vi "簡單狀態機.vi"() -> ()   [LabVIEW 2021]
panel:
  out "震幅":string
  out "頻率":string
  out "Waveform Graph":dbl[](graph)
  in  "Next Button":bool
  in  "Save Button":bool
  in  "Open Button":bool
  in  "Stop Button":bool
  in  "Cancel Button":bool
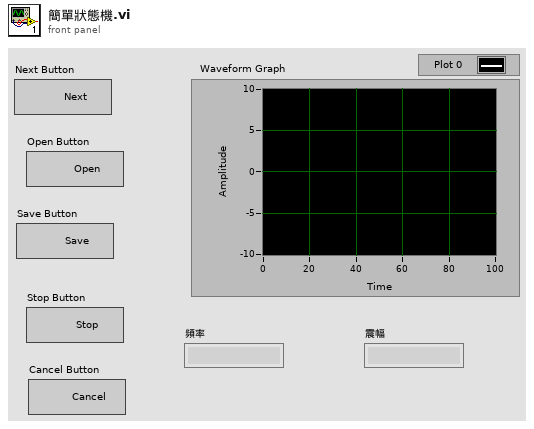
[diagram p1: front panel]
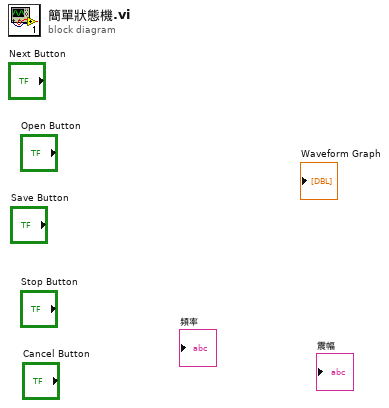
[diagram p0: block diagram]
diagram:
